vi "Voltech PM1000+ Ballast Measurement.vi"() -> ()   [LabVIEW 2015]
doc: "The purpose of this vi is to show the basic measurements that PM1000+ can make. The results are returned using the FRD command. This returns the results that are shown on the screen, in the order in which they appear on the screen. As results are selected using comms, the results are added to the bottom of the list, with the exception of harmonics, which always appear at the end of the list."
uses:
  <vilib>/Utility/error.llb/DialogType.ctl
  <instrlib>/Voltech PM1000+/Public/Configure/Configure Measurements (Ballast).vi
  <instrlib>/Voltech PM1000+/Voltech PM1000+.lvlib
panel:
  in  "Measurements":T1={"Voltage Harmonics"={"Range (7)"=7.0, "Sequence (Odd & Even)"=0}, "Current Harmonics"={"Range (7)"=7.0, "Sequence (Odd & Even)"=0}, "Measurements - Ballast"=[0, 1, 2, 5, 6]} {"Current Harmonics"."Sequence (Odd & Even)" items=["Odd & Even", "Odd Only"]; "Current Harmonics"."Range (7)" min=1.0 max=50.0 step=1.0; "Voltage Harmonics"."Sequence (Odd & Even)" items=["Odd & Even", "Odd Only"]; "Voltage Harmonics"."Range (7)" min=1.0 max=50.0 step=1.0}
  in  "Serial Configuration":T2={"Baud Rate"=19200, "Parity"=0, "Data Bits"=8, "Stop Bits"=10, "Flow Control"=2} {"Flow Control" items=["None"=0, "RTS/CTS"=2]; "Stop Bits" items=["1.0"=10]; "Data Bits" items=["8"=8]; "Parity" items=["None"]; "Baud Rate" items=["9600"=9600, "19200"=19200, "38400"=38400]}
  out "Number of Measurements Taken":u32
  out "error out":errorcluster
  in  "error in (no error)":errorcluster
  in  "Do ID Query":bool=TRUE
  in  "Do *RST":bool=TRUE
  in  "Select Mode (Normal)":u16(ring)=1 items=["Normal", "Ballast", "Inrush", "Standby Power", "Integrator"]
  in  "Enable Autozero  (True)":bool=TRUE caption="Autozero  (Enable)"
  in  "Enable Blanking (True)":bool=TRUE
  in  "Shunt (Internal)":u16(ring) items=["Internal", "External"]
  in  "Freq Source (Voltage)":u16(ring) items=["Voltage", "Current"]
  in  "Fixed/Auto Ranging":T3 {"Volts Ranging (Auto)" items=["Auto", "10Vpk", "46Vpk", "215Vpk", "900Vpk"]; "Amps Ranging (Auto)" items=["Auto", "0.1Apk", "0.4Apk", "1.6Apk", "6.25Apk", "25Apk", "100Apk"]}
  in  "Scaling":T4={"Voltage Sacling (1.0000)"=1.0, "Current Sacling (1.0000)"=1.0} {"Current Sacling (1.0000)" min=1e-06 max=1000000.0 step=1.0 format="%.6f"; "Voltage Sacling (1.0000)" min=1e-06 max=1000000.0 step=1.0 format="%.6f"}
  in  "VISA resource name":refnum<visa-resource-name>
  in  "stop":bool
  out "Parameter":string[](array[string])
  out "Value":dbl[](array[numeric])
  # "(c) 2008-2009 Voltech Instruments.  ALL RIGHTS RESERVED."
  # "Configuration Side"
  # "1. Leave it as default or set up the PM1000+ instruments on the left  \n    \"Configuration Side\".\n2. Press Ctrl+R to run the test.\n3. Press the lower right side \"STOP\" button to stop the test."
  # "1~50"
  # "1~50"
  # "Results Side"
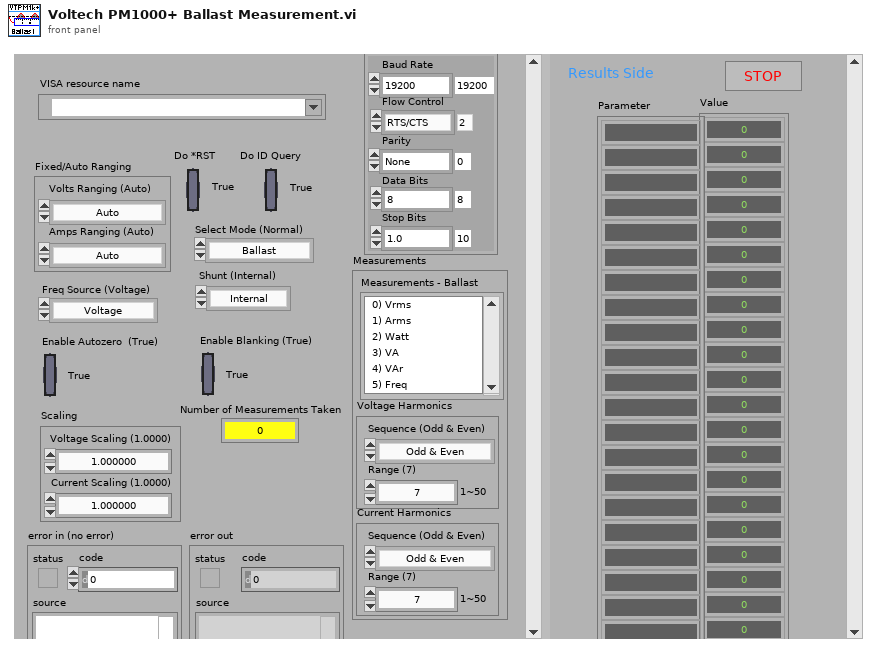
[diagram p1: front panel]
types:
  T1 = cluster{"Voltage Harmonics":cluster{"Range (7)":dbl, "Sequence (Odd & Even)":u16}, "Current Harmonics":cluster{"Range (7)":dbl, "Sequence (Odd & Even)":u16}, "Measurements - Ballast":i32[]}
  T2 = cluster{"Baud Rate":u32, "Parity":u16, "Data Bits":u16, "Stop Bits":u16, "Flow Control":u16}
  T3 = cluster{"Amps Ranging (Auto)":u16, "Volts Ranging (Auto)":u16}
  T4 = cluster{"Voltage Sacling (1.0000)":dbl, "Current Sacling (1.0000)":dbl}
  T5 = typedef "DialogType.ctl" = u16
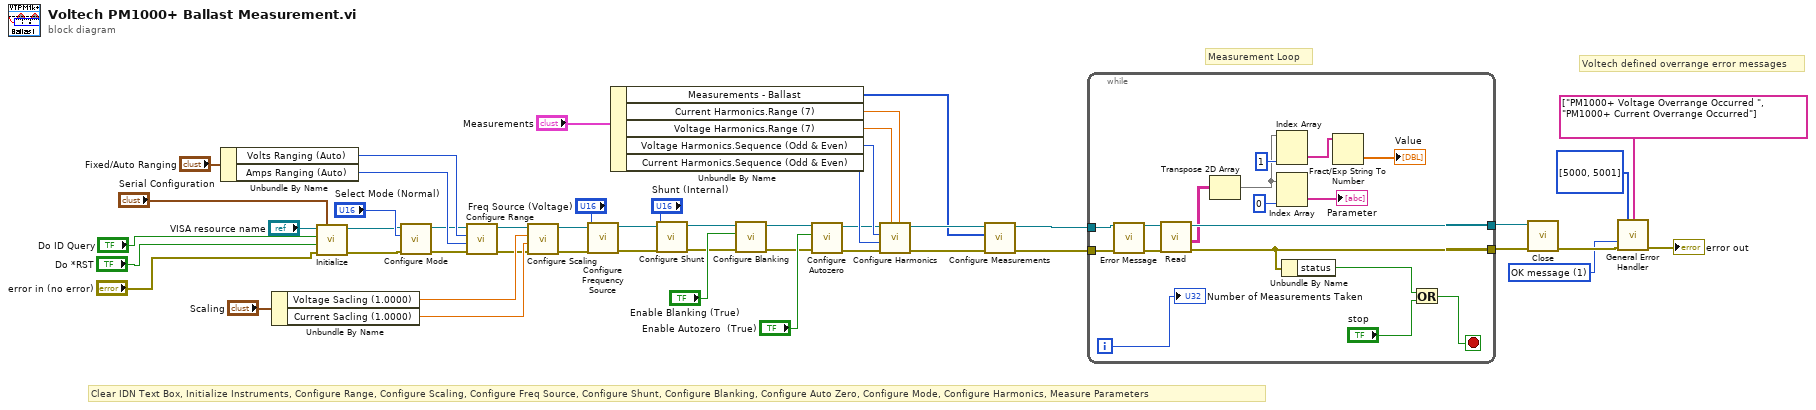
[diagram p0: block diagram]
diagram:
  w17 = T5 1 items=["no dialog", "OK message", "continue or stop message", "OK message + warnings", "continue/stop + warnings"] ("type of dialog (OK msg:1)")
  # "Voltech defined overrange error messages"
  # "Measurement Loop"
  # "Clear IDN Text Box, Initialize Instruments, Configure Range, Configure Scaling, Configure Freq Source, Configure Shunt, Configure Blanking, Configure Auto Zero, Configure Mode, Configure Harmonics, Measure Parameters"
  n1 = Unbundle By Name("Fixed/Auto Ranging") -> ("Volts Ranging (Auto)"=w41:u16, "Amps Ranging (Auto)"=w40:u16)
  n2 = Unbundle By Name("Scaling") -> ("Voltage Sacling (1.0000)"=w44:dbl, "Current Sacling (1.0000)"=w43:dbl)
  n3 = call <instrlib>:"Initialize.vi"("Serial Configuration"="Serial Configuration", "error in (no error)"="error in (no error)", "Reset (True)"="Do *RST", "ID Query (True)"="Do ID Query", "VISA resource name"="VISA resource name") -> ("error out"=w5:errorcluster, "VISA resource name out"=w6:refnum<visa-resource-name>)  [unwired: 5 in]
  n4 = call <instrlib>:"Configure Mode.vi"("error in (no error)"=w5, "Select Mode (Normal)"="Select Mode (Normal)", "VISA resource name"=w6) -> ("error out"=w11:errorcluster, "VISA resource name out"=w12:refnum<visa-resource-name>)  [unwired: 7 in]
  n5 = call <instrlib>:"Configure Range.vi"("error in (no error)"=w11, "Current Range (Auto)"=w40, "Voltage Range (Auto)"=w41, "VISA resource name"=w12) -> ("error out"=w9:errorcluster, "VISA resource name out"=w10:refnum<visa-resource-name>)  [unwired: 6 in]
  n6 = call <instrlib>:"Configure Scaling.vi"("error in (no error)"=w9, "Current Sacling (1.0000)"=w43, "Voltage Sacling (1.0000)"=w44, "VISA resource name"=w10) -> ("error out"=w46:errorcluster, "VISA resource name out"=w47:refnum<visa-resource-name>)  [unwired: 6 in]
  n7 = call <instrlib>:"Configure Frequency Source.vi"("error in (no error)"=w46, "Frequency Source (Voltage)"="Freq Source (Voltage)", "VISA resource name"=w47) -> ("error out"=w49:errorcluster, "VISA resource name out"=w48:refnum<visa-resource-name>)  [unwired: 7 in]
  n8 = Unbundle By Name("Measurements") -> ("Measurements - Ballast"=w34:i32[], "Current Harmonics.Range (7)"=w38:dbl, "Voltage Harmonics.Range (7)"=w37:dbl, "Voltage Harmonics.Sequence (Odd & Even)"=w33:u16, "Current Harmonics.Sequence (Odd & Even)"=w32:u16)
  n9 = call <instrlib>:"Configure Shunt.vi"("error in (no error)"=w49, "Shunt (Internal)"="Shunt (Internal)", "VISA resource name"=w48) -> ("error out"=w24:errorcluster, "VISA resource name out"=w23:refnum<visa-resource-name>)  [unwired: 7 in]
  n10 = call <instrlib>:"Configure Blanking.vi"("error in (no error)"=w24, "Enable Blanking (True)"="Enable Blanking (True)", "VISA resource name"=w23) -> ("error out"=w21:errorcluster, "VISA resource name out"=w22:refnum<visa-resource-name>)  [unwired: 7 in]
  n11 = call <instrlib>:"Configure Autozero.vi"("error in (no error)"=w21, "Enable Autozero (True)"="Enable Autozero  (True)", "VISA resource name"=w22) -> ("error out"=w13:errorcluster, "VISA resource name out"=w14:refnum<visa-resource-name>)  [unwired: 7 in]
  n12 = call <instrlib>:"Configure Harmonics.vi"("Current Harmonic Range (7)"=w38, "Voltage Harmonic Range (7)"=w37, "error in (no error)"=w13, "Current Harmonic Sequence (Odd & Even)"=w32, "Voltage Harmonic Sequence (Odd & Even)"=w33, "VISA resource name"=w14) -> ("error out"=w35:errorcluster, "VISA resource name out"=w36:refnum<visa-resource-name>)  [unwired: 4 in]
  n13 = call-poly <instrlib>:"Configure Measurements.vi"("error in (no error)"=w35, "Ballast Measurements"=w34, "VISA resource name"=w36) -> ("error out"=w28:errorcluster, "VISA resource name out"=w29:refnum<visa-resource-name>)  [unwired: 7 in]
  n14 = while {
    tunnel: w29 -> [w55]
    tunnel: w28 -> [w54]
    tunnel: [w66] -> w27
    tunnel: [w53] -> w26
    i -> [w65]
    stop <- w52 stop-if-true
    n15 = call <instrlib>:"Error Message.vi"("VISA resource name"=w55, "error in (no error)"=w54) -> ("VISA resource name out"=w57:refnum<visa-resource-name>, "error out"=w56:errorcluster)  [unwired: 12 in]
    n16 = call <instrlib>:"Read.vi"("error in (no error)"=w56, "VISA resource name"=w57) -> ("error out"=w53:errorcluster, "Measurement Results"=w62:string[][], "VISA resource name out"=w66:refnum<visa-resource-name>)  [unwired: 7 in]
    n17 = Transpose 2D Array(2D array=w62) -> (transposed array=w61:string[][])
    n18 = Index Array(array=w61, index (col)=1) -> (element=w59:string[])  [unwired: 1 in]
    n19 = Index Array(array=w61, index (col)=0) -> (element=→"Parameter":string[])  [unwired: 1 in]
    n20 = Unbundle By Name(w53) -> ("status"=w50:bool)
    n21 = Fract/Exp String To Number(string=w59) -> (number=→"Value":dbl[])  [unwired: 3 in, 1 out]
    n22 = Or(x=w50, y="stop") -> (x .or. y?=w52:bool)
    "Number of Measurements Taken" <- w65
  }
  n23 = call <instrlib>:"Close.vi"("error in (no error)"=w26, "VISA resource name"=w27) -> ("error out"=w18:errorcluster)  [unwired: 9 in]
  n24 = call <vilib>:"General Error Handler.vi"("[user-defined codes]"=i32[] [5000, 5001], "[user-defined descriptions]"=string[] ["PM1000+ Voltage Overrange Occurred ", "PM1000+ Current Overrange Occurred"], "type of dialog (OK msg:1)"=w17, "error in (no error)"=w18) -> ("error out"=→"error out":errorcluster)  [unwired: 7 in, 4 out]
